vi "set_x_resolution.vi"(8 "error in (no error)":errorcluster, 10 "x resolution":i32, 11 "TrajectoryAK101022Resonance in":refnum<class "TrajectoryAK101022Resonance.lvclass">) -> (0 "error out":errorcluster, 3 "TrajectoryAK101022Resonance out":refnum<class "TrajectoryAK101022Resonance.lvclass">)   [LabVIEW 2010, in "TrajectoryAK101022Resonance.lvclass"]
uses:
  TrajectoryAK101022Resonance.lvclass
  TrajectoryAK101022Resonance.lvclass/TrajectoryAK101022Resonance.ctl
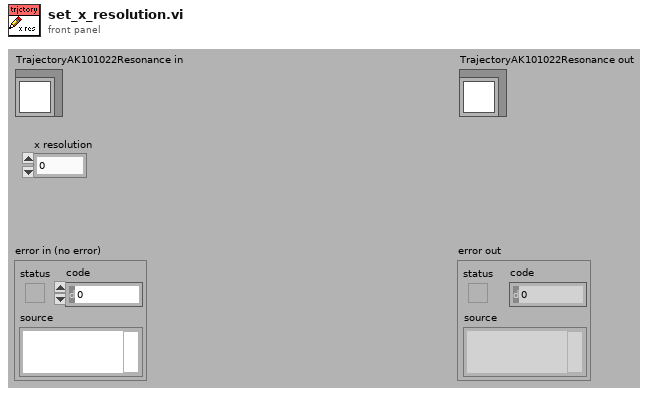
[diagram p1: front panel]
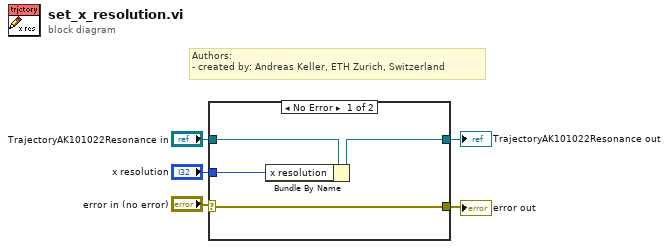
[diagram p0: block diagram]
diagram:
  # "Authors: \n- created by: Andreas Keller, ETH Zurich, Switzerland"
  n1 = case shown="No Error" "error in (no error)" {
    selector: "error in (no error)" -> [w9 w10]
    tunnel: [w9 w10] -> w4
    tunnel: "TrajectoryAK101022Resonance in" -> [w7 w11]
    tunnel: [w8 w11] -> w2
    tunnel: "x resolution" -> [w6 _]
    frame No Error {
      n2 = Bundle By Name(cluster=w7, "x resolution"=w6) -> (w8:refnum<class "TrajectoryAK101022Resonance.lvclass">)
    }
    frame Error {
    }
  }
  "TrajectoryAK101022Resonance out" <- w2
  "error out" <- w4
